vi "MCL C Focus Get Focus Mode.vi"(10 "handle":i32, 11 "focusLocked":i32) -> (2 "function return":i32, 3 "focusLocked out":i32)   [LabVIEW 2017, in "Madlib.lvlib"]
doc: "MADLIB_API int MCL_CFocusGetFocusMode(int *focusLocked, int handle);"
uses:
  Madlib.lvlib
  Madlib.dll
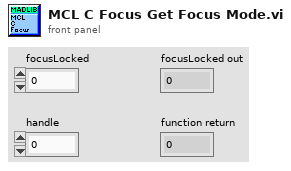
[diagram p1: front panel]
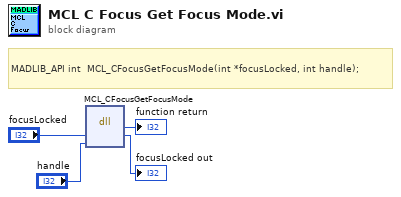
[diagram p0: block diagram]
diagram:
  # "MADLIB_API\tint\t\tMCL_CFocusGetFocusMode(int *focusLocked, int handle);"
  n1 = dll-call lib="C:/Users/francesco/dev/pump-probe/Piezo/lvlib/Madlib.*" fn="MCL_CFocusGetFocusMode"("focusLocked"="focusLocked", "handle"="handle") -> (→"function return":i32, "focusLocked"=→"focusLocked out":i32)  [unwired: 4 in, 2 out]
